vi "GEA2 Read ERD Multiple Messages.vi"(0 "GEA2 Reference In":refnum<k24>, 1 "Retry Count":i32=5, 2 "Read Timeout (ms)":u32=500, 5 "GEA Inputs":T3 {"Destination" format="%.0x"; "Source" format="%.0x"}, 7 "Read ERD List":T2[](array[typedef]) {"ERD Number" format="%.0x"}, 9 "Expected Command 2":string=".*", 10 "Expected Data 2":string, 11 "Error In":errorcluster, 12 "#ERDs per message":i32=1 min=1 step=1, 13 "Verify ERD Response?":bool=TRUE, 14 "Disable Expected Data":bool) -> (4 "GEA2 Reference Out":refnum<k24>, 6 "Raw Data Out":string[](array[string]), 8 "ERD Data Out":T1[](array[typedef]) {"ERD Number" format="%.0x"}, 15 "Error Out":errorcluster)   [LabVIEW 2014, in "GEA2_Toolkit.lvlib"]
uses:
  library/GEA2_Toolkit.lvlib
  C:/Automation/DLLs/PC Tools .NET/GeaCommunication.dll
  Automation/DLLs/PC Tools .NET/GeaCommunication.dll
  type defs/Source_Destination.ctl
  type defs/ERD Read Data In.ctl
  type defs/ERD Read Data Out.ctl
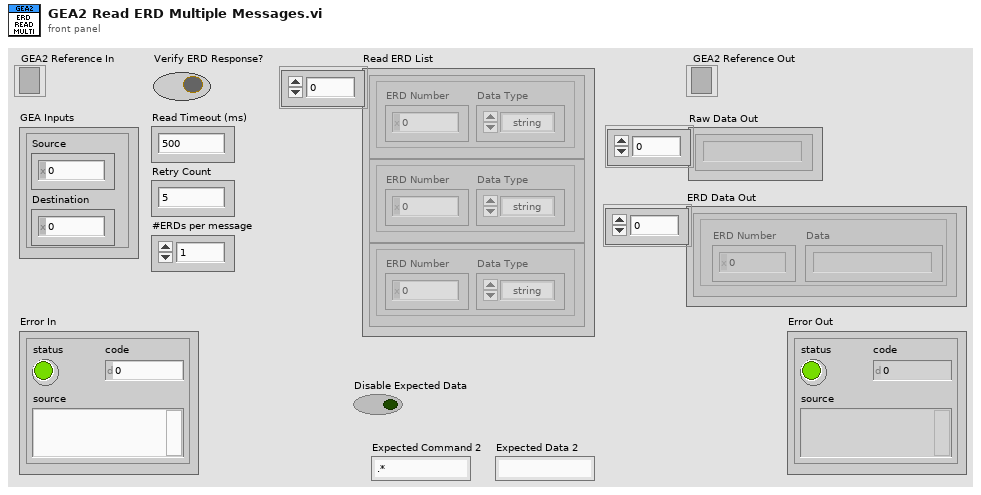
[diagram p1: front panel]
types:
  T1 = typedef "GEA2_Toolkit.lvlib/ERD Read Data Out.ctl" = cluster{"ERD Number":u16, "Data":string}
  T2 = typedef "GEA2_Toolkit.lvlib/ERD Read Data In.ctl" = cluster{"ERD Number":u16, "Data Type":enum16{"string", "boolean", "uint8_t", "uint16_t", "uint32_t", "uint64_t"}}
  T3 = typedef "GEA2_Toolkit.lvlib/Source_Destination.ctl" = cluster{"Source":u8, "Destination":u8}
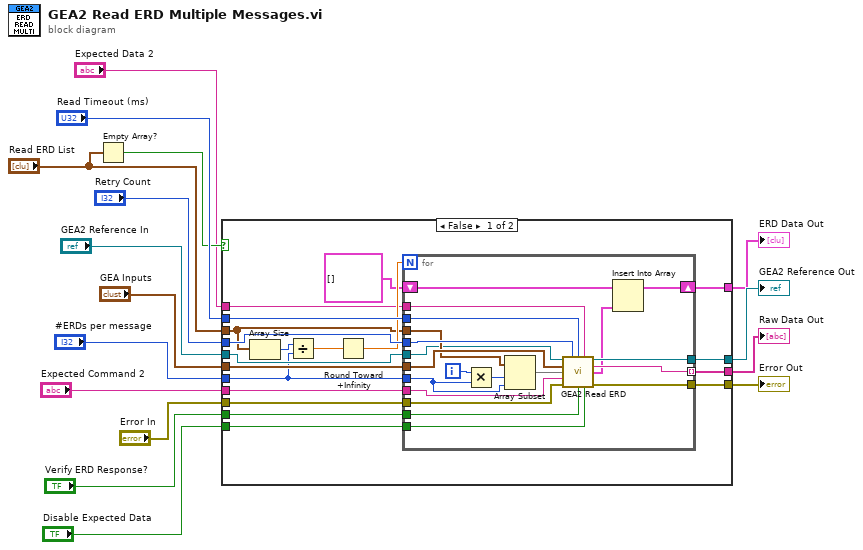
[diagram p0: block diagram]
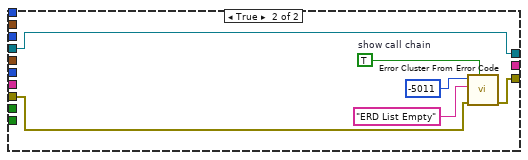
[diagram p2: hidden frame]
diagram:
  n1 = Empty Array?(array="Read ERD List") -> (empty?=w4:bool)
  n2 = case shown="False" w4 {
    tunnel: [w35 w56] -> w16
    tunnel: "Error In" -> [w34 w58]
    tunnel: [w33 w57] -> w14
    tunnel: "Verify ERD Response?" -> [w32 _]
    tunnel: "GEA Inputs" -> [w31 _]
    tunnel: "Read Timeout (ms)" -> [w30 _]
    tunnel: "Retry Count" -> [w29 _]
    tunnel: "GEA2 Reference In" -> [w28 w56]
    tunnel: "#ERDs per message" -> [w24 _]
    tunnel: [w23 _] -> w7
    tunnel: [w21 _] -> w6
    tunnel: "Read ERD List" -> [w20 _]
    tunnel: "Expected Command 2" -> [w19 _]
    tunnel: "Disable Expected Data" -> [w18 _]
    tunnel: "Expected Data 2" -> [w17 _]
    frame False {
      n3 = Array Size(array=w20) -> (size(s)=w27:i32)
      n4 = Divide(x=w27, y=w24) -> (x/y=w26:dbl)
      n5 = Round Toward +Infinity(x=w26) -> (ceil(x): smallest int >= x=w25:dbl)
      n6 = for {
        N: w25 -> [_]
        tunnel: w32 -> [w52]
        tunnel: w31 -> [w51]
        tunnel: [w50] -> w23 mode=indexing
        tunnel: w30 -> [w49]
        tunnel: w29 -> [w48]
        tunnel: w20 -> [w47]
        tunnel: w24 -> [w46]
        shift-right: [w39] -> w21
        shift-left: T1[] [] -> [w41]
        tunnel: w34 -> [w54]
        tunnel: [w53] -> w33
        tunnel: w28 -> [w43]
        tunnel: [w55] -> w35
        tunnel: w19 -> [w38]
        tunnel: w18 -> [w37]
        tunnel: w17 -> [w36]
        i -> [w45]
        n7 = Multiply(x=w45, y=w46) -> (x*y=w44:i32)
        n8 = Array Subset(array=w47, index=w44, length=w46) -> (w42:T2[])
        n9 = call "GEA2 Read ERD.vi"("GEA2 Reference In"=w43, "Retry Count"=w48, "Read Timeout (ms)"=w49, "Expected Data 2"=w36, "GEA Inputs"=w51, "Read ERD List"=w42, "Expected Command 2"=w38, "Error In"=w54, "Verify ERD Response?"=w52, "Disable Expected Data"=w37) -> ("GEA2 Reference Out"=w55:refnum<k24>, "Raw Data Out"=w50:string, "ERD Data Out"=w40:T1[], "Error Out"=w53:errorcluster)  [unwired: 2 in]
        n10 = Insert Into Array(array=w41, new element=w40) -> (w39:T1[])  [unwired: 1 in]
      }
    }
    frame True {
      w59 = TRUE  # show call chain
      n11 = call <vilib>:"Error Cluster From Error Code.vi"("show call chain? (False)"=w59, "error in (no error)"=w58, "error message (\"\")"="ERD List Empty" ("error message (\"\")"), "error code (0)"=-5011) -> ("error out"=w57:errorcluster)  [unwired: 5 in]
    }
  }
  "GEA2 Reference Out" <- w16
  "Error Out" <- w14
  "Raw Data Out" <- w7
  "ERD Data Out" <- w6
